vi "Main.vi"(8 "error in":errorcluster, 11 "Cascade512II in":refnum<class "DAQCascade512II.lvclass">) -> (0 "error out":errorcluster, 3 "component":refnum<class "DAQCascade512II.lvclass">)   [LabVIEW 2012, in "DAQCascade512II.lvclass"]
doc: "Main VI of the component. This should contain the GUI of your component and be called when creating an executable."
uses:
  DAQCascade512II.lvclass
  setting cluster.ctl
  DAQCascade512II.lvclass/DAQCascade512II.ctl
  <vilib>/Distrio/Murmex/InitialiseMessage/InitialiseMessage.lvclass
  <vilib>/Distrio/Murmex/Murmex/update_cluster.ctl
  <vilib>/Distrio/Murmex/TerminateMessage/TerminateMessage.lvclass
  <vilib>/Distrio/Murmex/ConfigureMessage/ConfigureMessage.lvclass
  <vilib>/Distrio/Murmex/StartMessage/StartMessage.lvclass
  <vilib>/Distrio/Murmex/StartMessage/run mode enum.ctl
  <vilib>/Distrio/Murmex/Murmex/Set configure at initialise.vi
  <vilib>/Distrio/Murmex/Murmex/Set log reference.vi
  <vilib>/Distrio/Murmex/Murmex/Set VI reference.vi
  <vilib>/Distrio/Murmex/Murmex/Set relay start stop to observers.vi
  <vilib>/Distrio/Murmex/Murmex/Murmex.lvclass
panel:
  in  "Button: configuration":bool
  in  "buttom:quit":bool
  in  "terminate?":bool
  in  "Tab Control":enum32{"Acqusition", "Debug"}(tab)
  in  "switch:focus/acqurie":bool
  out "saved frames":dbl
  in  "setting":T1={"Exposure (sec)"=0.1, "no. of frames"=2, "File Path"=path ""} {"Exposure (sec)" format="%.3f"}
  in  "2x2 binning":bool
  in  "Button:cancel process":bool
  in  "button: start":bool
  in  "Log":string
  in  "ID":string
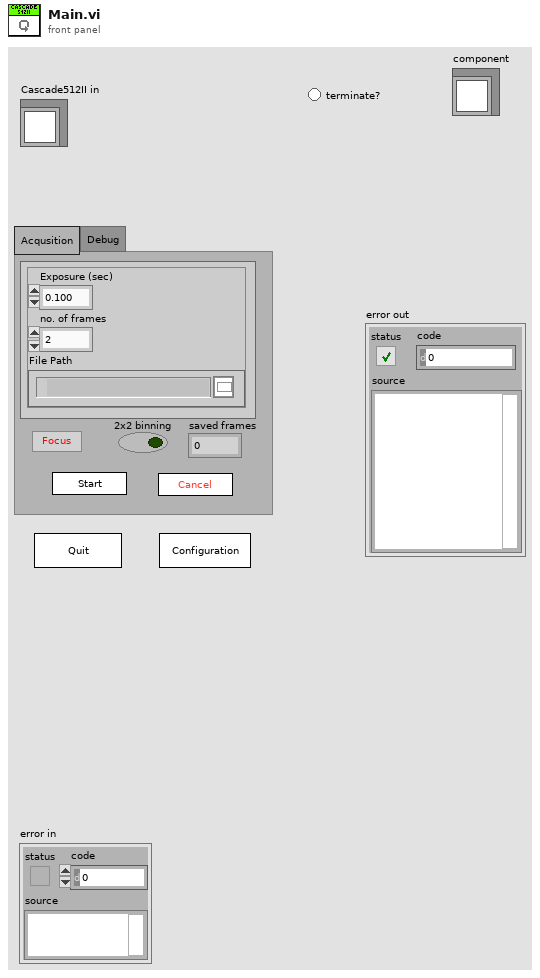
[diagram p1: front panel]
types:
  T1 = typedef "DAQCascade512II.lvclass/setting cluster.ctl" = cluster{"Exposure (sec)":dbl, "no. of frames":u32, "File Path":path}
  T2 = typedef "Murmex.lvlib/Murmex.lvclass/update_cluster.ctl" = cluster{"target ID":string, "key chains":string[], "values":variant[]}
  T3 = typedef "Murmex.lvlib/StartMessage.lvclass/run mode enum.ctl" = enum16{"infinite", "finite"}
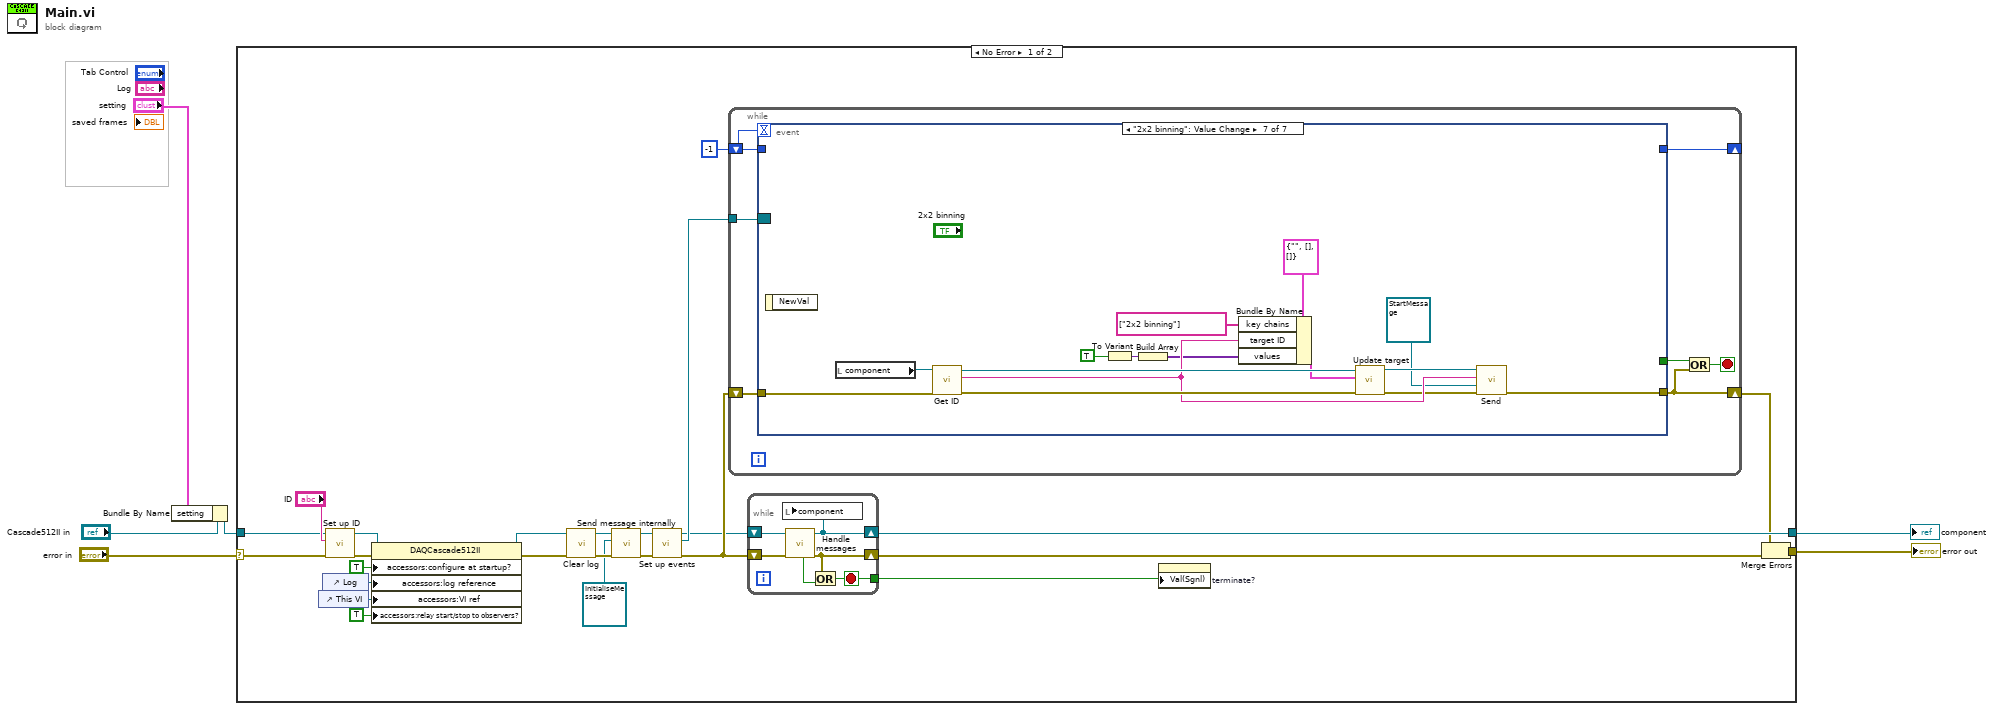
[diagram p0: block diagram]
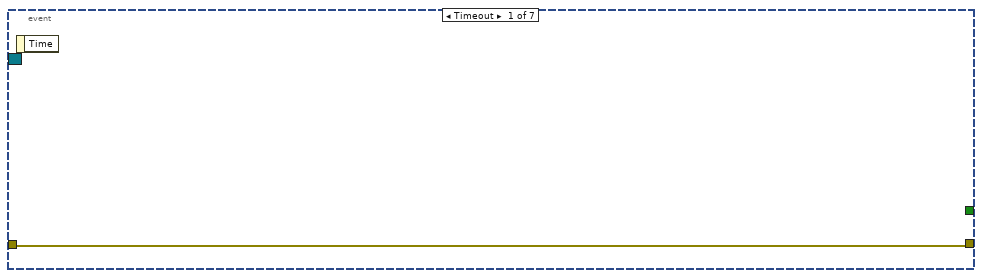
[diagram p2: hidden frame]
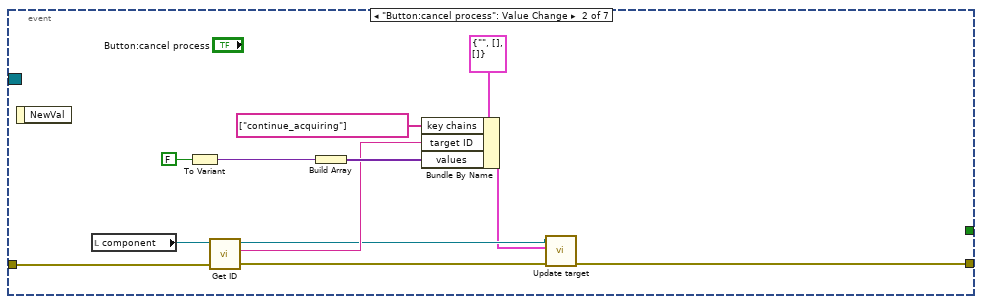
[diagram p3: hidden frame]
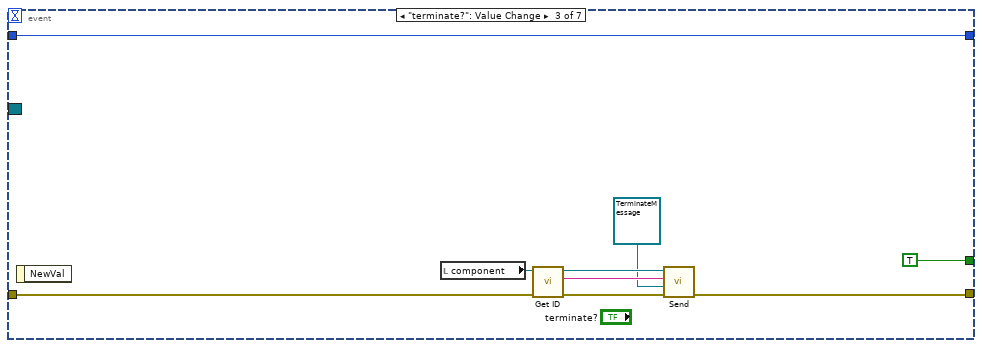
[diagram p4: hidden frame]
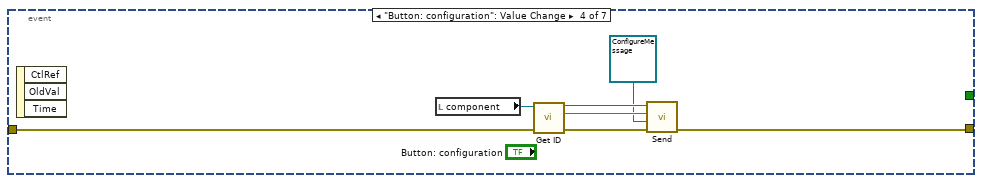
[diagram p5: hidden frame]
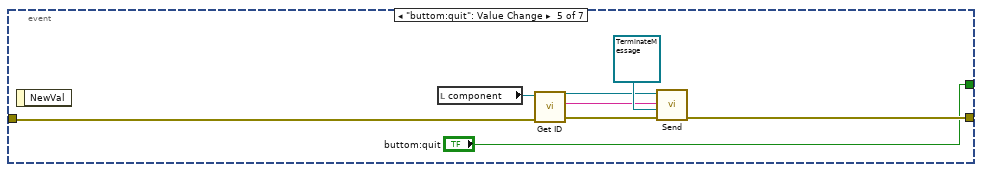
[diagram p6: hidden frame]
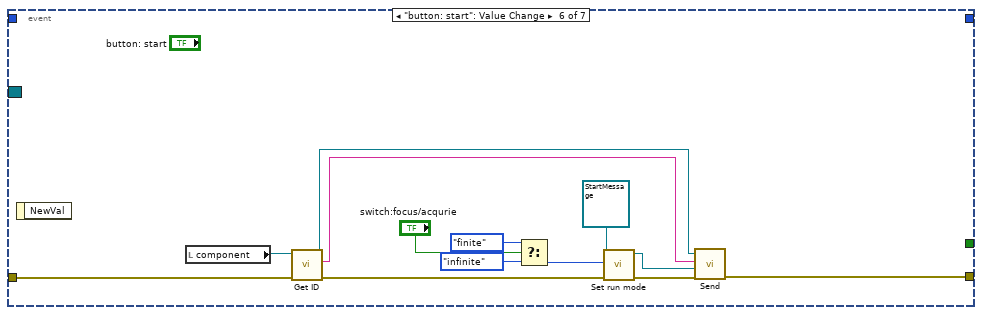
[diagram p7: hidden frame]
diagram:
  n1 = Bundle By Name(cluster="Cascade512II in", "setting"="setting") -> (w2:refnum<class "DAQCascade512II.lvclass">)
  n2 = case shown="No Error" "error in" {
    selector: "error in" -> [w8 w109]
    tunnel: [w31 w110] -> w6
    tunnel: [w16 w109] -> w4
    tunnel: w2 -> [w9 w110]
    frame No Error {
      n3 = control-ref of="This VI"() -> (w28:refnum<vi>)
      n4 = control-ref of="Log"() -> (w29:refnum<vi>)
      n5 = call <vilib>:"Set up ID.vi"("error in (no error)"=w8, "component ID"="ID", "MurmexBase in"=w9) -> ("error out"=w26:errorcluster, "MurmexBase out"=w25:refnum<class "DAQCascade512II.lvclass">)  [unwired: 6 in, 1 out]
      n6 = property class="DAQCascade512II"(reference=w25, error in=w26, "accessors:configure at startup?"=TRUE ("configure at startup?"), "accessors:log reference"=w29, "accessors:VI ref"=w28, "accessors:relay start/stop to observers?"=TRUE ("relay start/stop to observers?")) -> (reference out=w24:refnum<class "DAQCascade512II.lvclass">, error out=w23:errorcluster)
      n7 = call <vilib>:"Clear log.vi"("error in (no error)"=w23, "MurmexBase in"=w24) -> ("error out"=w21:errorcluster, "MurmexBase out"=w22:refnum<class "DAQCascade512II.lvclass">)  [unwired: 8 in]
      n8 = call <vilib>:"Send message internally.vi"("error in (no error)"=w21, "Message"=refnum<class "InitialiseMessage.lvclass"> refnum ("Distrio Murmex 1.5:InitialiseMessage"), "Murmex in"=w22) -> ("error out"=w14:errorcluster, "Murmex out"=w12:refnum<class "DAQCascade512II.lvclass">)  [unwired: 7 in]
      n9 = call <vilib>:"Set up events.vi"("error in (no error)"=w14, "MurmexBase in"=w12) -> ("error out"=w13:errorcluster, "Event Registration Refnum"=w11:refnum<event-registration>, "MurmexBase out"=w7:refnum<class "DAQCascade512II.lvclass">)  [unwired: 7 in]
      n10 = while {
        shift-right: [w36] -> w18
        shift-left: w13 -> [w38]
        tunnel: w11 -> [w32]
        shift-right: [w33] -> _
        shift-left: -1 -> [w34]
        stop <- w35 stop-if-true
        n11 = event shown="[6] \"2x2 binning\": Value Change" {
          selector: w32 -> [_ _ _ _ _ _ _]
          dyn-events: _ -> [_ _ _ _ _ _ _]
          timeout: w34 -> [_ _ _ _ _ _ _]
          tunnel: w38 -> [w39 w50 w55 w62 w69 w87 w99]
          tunnel: [w39 w42 w54 w61 w68 w84 w98] -> w36
          tunnel: [_ _ TRUE ("terminate?") _ "buttom:quit" _ _] -> w37
          tunnel: [_ _ w52 _ _ _ _] -> w33
          tunnel: w34 -> [_ _ w52 _ _ _ _]
          event Timeout {
            n12 = event-data() -> ()  [unwired: 1 in, 1 out]
          }
          event "Button:cancel process": Value Change {
            n13 = event-data() -> ()  [unwired: 1 in, 1 out]
            n14 = local read "component"() -> (w51:refnum<class "DAQCascade512II.lvclass">)
            n15 = To Variant(anything=FALSE) -> (Variant=w47:variant)
            n16 = call <vilib>:"Get ID.vi"("error in (no error)"=w50, "Murmex in"=w51) -> ("error out"=w43:errorcluster, "component id"=w45:string, "Murmex out"=w41:refnum<class "DAQCascade512II.lvclass">)  [unwired: 7 in]
            n17 = Build Array(w47) -> (w46:variant[])
            n18 = Bundle By Name(cluster=T2 {"target ID"="", "key chains"=[], "values"=[]} ("update cluster"), "key chains"=string[] ["continue_acquiring"], "target ID"=w45, "values"=w46) -> (w40:T2)
            n19 = call <vilib>:"Update target.vi"("error in (no error)"=w43, "update cluster"=w40, "MurmexBase in"=w41) -> ("error out"=w42:errorcluster)  [unwired: 7 in, 1 out]
          }
          event "terminate?": Value Change {
            n20 = event-data() -> ()  [unwired: 1 in, 1 out]
            n21 = local read "component"() -> (w59:refnum<class "DAQCascade512II.lvclass">)
            n22 = call <vilib>:"Get ID.vi"("error in (no error)"=w55, "Murmex in"=w59) -> ("error out"=w56:errorcluster, "component id"=w58:string, "Murmex out"=w57:refnum<class "DAQCascade512II.lvclass">)  [unwired: 7 in]
            n23 = call <vilib>:"Send.vi"("error in (no error)"=w56, "Message"=refnum<class "TerminateMessage.lvclass"> refnum ("Distrio Murmex 1.5:TerminateMessage"), "recipient"=w58, "Murmex in"=w57) -> ("error out"=w54:errorcluster)  [unwired: 6 in, 1 out]
          }
          event "Button: configuration": Value Change {
            n24 = event-data() -> ()  [unwired: 1 in, 3 out]
            n25 = local read "component"() -> (w66:refnum<class "DAQCascade512II.lvclass">)
            n26 = call <vilib>:"Get ID.vi"("Murmex in"=w66) -> ("component id"=w64:string, "Murmex out"=w65:refnum<class "DAQCascade512II.lvclass">)  [unwired: 8 in, 1 out]
            n27 = call <vilib>:"Send.vi"("error in (no error)"=w62, "Message"=refnum<class "ConfigureMessage.lvclass"> refnum ("Distrio Murmex 1.5:ConfigureMessage"), "recipient"=w64, "Murmex in"=w65) -> ("error out"=w61:errorcluster)  [unwired: 6 in, 1 out]
          }
          event "buttom:quit": Value Change {
            n28 = event-data() -> ()  [unwired: 1 in, 1 out]
            n29 = local read "component"() -> (w74:refnum<class "DAQCascade512II.lvclass">)
            n30 = call <vilib>:"Get ID.vi"("error in (no error)"=w69, "Murmex in"=w74) -> ("error out"=w70:errorcluster, "component id"=w71:string, "Murmex out"=w72:refnum<class "DAQCascade512II.lvclass">)  [unwired: 7 in]
            n31 = call <vilib>:"Send.vi"("error in (no error)"=w70, "Message"=refnum<class "TerminateMessage.lvclass"> refnum ("Distrio Murmex 1.5:TerminateMessage"), "recipient"=w71, "Murmex in"=w72) -> ("error out"=w68:errorcluster)  [unwired: 6 in, 1 out]
          }
          event "button: start": Value Change {
            n32 = event-data() -> ()  [unwired: 1 in, 1 out]
            n33 = local read "component"() -> (w86:refnum<class "DAQCascade512II.lvclass">)
            n34 = call <vilib>:"Get ID.vi"("error in (no error)"=w87, "Murmex in"=w86) -> ("error out"=w83:errorcluster, "component id"=w85:string, "Murmex out"=w80:refnum<class "DAQCascade512II.lvclass">)  [unwired: 7 in]
            n35 = Select(t=run_mode_enum."finite" ("run mode"), s="switch:focus/acqurie", f=run_mode_enum."infinite" ("run mode")) -> (s? t:f=w76:T3)
            n36 = call <vilib>:"Set run mode.vi"("error in (no error)"=w83, "run mode"=w76, "StartMessage in"=refnum<class "StartMessage.lvclass"> refnum ("Distrio Murmex 1.5:StartMessage")) -> ("error out"=w82:errorcluster, "StartMessage out"=w81:refnum<class "StartMessage.lvclass">)  [unwired: 7 in]
            n37 = call <vilib>:"Send.vi"("error in (no error)"=w82, "Message"=w81, "recipient"=w85, "Murmex in"=w80) -> ("error out"=w84:errorcluster)  [unwired: 6 in, 1 out]
          }
          event "2x2 binning": Value Change {
            n38 = event-data() -> ()  [unwired: 1 in, 1 out]
            n39 = local read "component"() -> (w102:refnum<class "DAQCascade512II.lvclass">)
            n40 = call <vilib>:"Get ID.vi"("error in (no error)"=w99, "Murmex in"=w102) -> ("error out"=w101:errorcluster, "component id"=w97:string, "Murmex out"=w100:refnum<class "DAQCascade512II.lvclass">)  [unwired: 7 in]
            n41 = To Variant(anything=TRUE ("2x2 binning")) -> (Variant=w93:variant)
            n42 = Build Array(w93) -> (w92:variant[])
            n43 = Bundle By Name(cluster=T2 {"target ID"="", "key chains"=[], "values"=[]} ("update cluster"), "key chains"=string[] ["2x2 binning"], "target ID"=w97, "values"=w92) -> (w94:T2)
            n44 = call <vilib>:"Update target.vi"("error in (no error)"=w101, "update cluster"=w94, "MurmexBase in"=w100) -> ("error out"=w91:errorcluster, "MurmexBase out"=w90:refnum<class "DAQCascade512II.lvclass">)  [unwired: 7 in]
            n45 = call <vilib>:"Send.vi"("error in (no error)"=w91, "Message"=refnum<class "StartMessage.lvclass"> refnum ("Distrio Murmex 1.5:StartMessage"), "recipient"=w97, "Murmex in"=w90) -> ("error out"=w98:errorcluster)  [unwired: 6 in, 1 out]
          }
        }
        n46 = Or(x=w37, y=w36) -> (x .or. y?=w35:bool)
      }
      n47 = while {
        shift-right: [w103] -> w31
        shift-left: w7 -> [w107]
        shift-right: [w105] -> w17
        shift-left: w13 -> [w108]
        tunnel: [w104] -> w19
        stop <- w104 stop-if-true
        n48 = call <vilib>:"Handle messages.vi"("error in (no error)"=w108, "Murmex in"=w107) -> ("error out"=w105:errorcluster, "Murmex out"=w103:refnum<class "DAQCascade512II.lvclass">, "terminated?"=w106:bool)  [unwired: 7 in]
        n49 = local write "component"(w103) -> ()
        n50 = Or(x=w105, y=w106) -> (x .or. y?=w104:bool)
      }
      n51 = property on="terminate?" class="Bool"("Val(Sgnl)"=w19) -> ()  [unwired: 2 in, 2 out]
      n52 = Merge Errors(w18, w17) -> (w16:errorcluster)
    }
    frame Error {
    }
  }
  "component" <- w6
  "error out" <- w4
